vi "myRIO_BRig_Host_endExp_storeFile.vi"(10 "input_expPrefix":string, 11 "input_fileName":string) -> (1 "output_Iexist_stored":bool, 2 "output_Iexist_orig":bool)   [LabVIEW 2014]
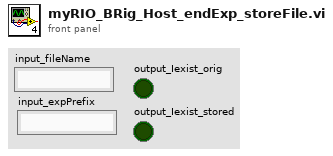
[diagram p1: front panel]
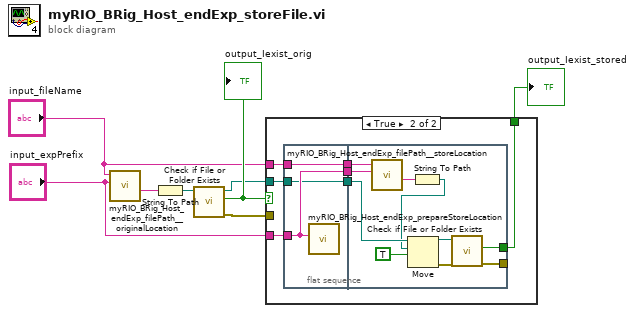
[diagram p0: block diagram]
diagram:
  n1 = call "myRIO_BRig_Host_endExp_filePath__originalLocation.vi"("input_expPrefix"="input_expPrefix", "input_fileName"="input_fileName") -> ("output_filePath"=w4:string)  [unwired: 9 in]
  n2 = String To Path(string=w4) -> (path=w8:path)
  n3 = call <vilib>:"Check if File or Folder Exists.vi"("path"=w8) -> ("error out"=w6:errorcluster, "file or folder exists?"=w7:bool, "dup path"=w5:path)  [unwired: 8 in]
  "output_Iexist_orig" <- w7
  n4 = case shown="True" w7 {
    tunnel: w6 -> [_ _]
    tunnel: w5 -> [_ w10]
    tunnel: "input_expPrefix" -> [_ w15]
    tunnel: "input_fileName" -> [_ w13]
    tunnel: [_ w9] -> w1
    frame False {
    }
    frame True {
      n5 = flat-sequence {
        tunnel: w15 -> [w17]
        tunnel: [w18] -> w14
        tunnel: w13 -> [w18]
        tunnel: [w17] -> w12
        tunnel: [w16] -> w11
        tunnel: w10 -> [w16]
        tunnel: w14 -> [w28]
        tunnel: w12 -> [w27]
        tunnel: w11 -> [w22]
        tunnel: [w20] -> w9
        tunnel: [w19] -> _
        frame #0 {
          n6 = call "myRIO_BRig_Host_endExp_prepareStoreLocation.vi"("input_expPrefix"=w17) -> ()  [unwired: 10 in, 1 out]
        }
        frame #1 {
          n7 = call "myRIO_BRig_Host_endExp_filePath__storeLocation.vi"("input_fileName"=w27, "input_filePath_storage"=w28) -> ("output_filePath"=w26:string)  [unwired: 9 in]
          n8 = String To Path(string=w26) -> (path=w21:path)
          n9 = Move(source path=w22, 9:TRUE ("overwrite (F)"), 10:w21) -> (error out=w23:errorcluster, 3:w24:path)  [unwired: 2 in, 1 out]
          n10 = call <vilib>:"Check if File or Folder Exists.vi"("error in (no error)"=w23, "path"=w24) -> ("error out"=w19:errorcluster, "file or folder exists?"=w20:bool)  [unwired: 7 in, 1 out]
        }
      }
    }
  }
  "output_Iexist_stored" <- w1
